vi "FPL-Compute FPL.vi"(0 "path in":path, 11 "error in (no error)":errorcluster) -> (4 "path out":path, 15 "error out":errorcluster)   [LabVIEW 2015]
uses:
  Utility VIs/Math VIs/Z to dB, degrees (1D).vi
panel:
  out "XY Graph":T1(graph)
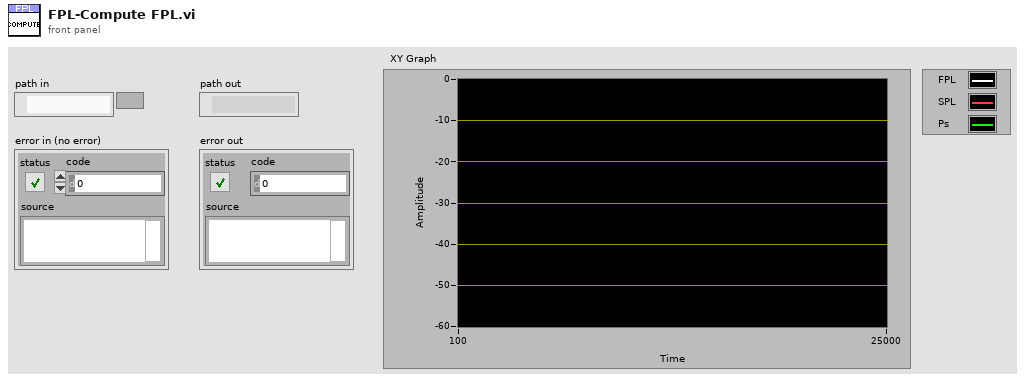
[diagram p1: front panel]
types:
  T1 = cluster{"Frequency (Hz)":dbl[], "Magnitude (dB)":dbl[]}[]
  T2 = cluster{"Frequency (Hz)":dbl[], "Magnitude (dB)":dbl[]}
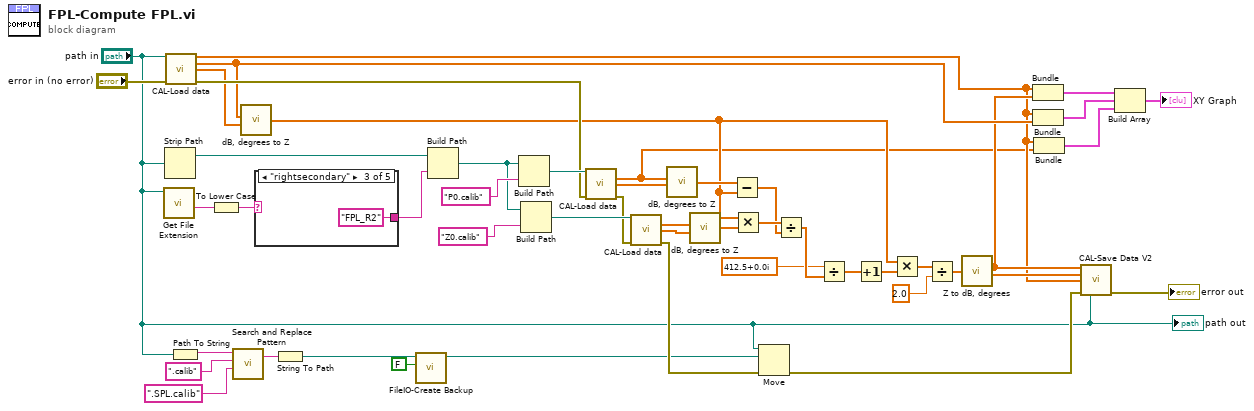
[diagram p0: block diagram]
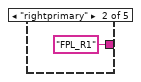
[diagram p3: hidden frame]
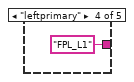
[diagram p4: hidden frame]
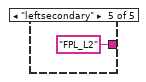
[diagram p5: hidden frame]
diagram:
  n1 = call <vilib>:"Get File Extension.vi"("file"="path in") -> ("filename without extension"=w48:string)  [unwired: 6 in, 4 out]
  n2 = Strip Path(path="path in") -> (stripped path=w46:path)  [unwired: 1 out]
  n3 = call "CAL-Load data.vi"("user path"="path in", "error in (no error)"="error in (no error)") -> ("Frequency (Hz)"=w4:dbl[], "Mag"=w18:dbl[], "Phase"=w33:dbl[], "error out"=w38:errorcluster)  [unwired: 6 in, 4 out]
  n4 = Path To String(path="path in") -> (string=w16:string)
  n5 = To Lower Case(string=w48) -> (all lower case string=w47:string)
  n6 = call <vilib>:"Search and Replace Pattern.vi"("string"=w16, "regular expression (\"\")"=".calib" ("regular expression (\"\")"), "replace string (\"\")"=".SPL.calib" ("regular expression (\"\")")) -> ("result string"=w13:string)  [unwired: 2 in, 1 out]
  n7 = call "dB, degrees to Z.vi"("Magnitude (dB)"=w18, "Phase (degrees)"=w33) -> ("Z"=w21:cdb[])  [unwired: 5 in]
  n8 = case shown="\"rightsecondary\"" w47 {
    tunnel: [_ "FPL_R1" "FPL_R2" "FPL_L1" "FPL_L2"] -> w45
    frame "", Default {
    }
    frame "rightprimary" {
    }
    frame "rightsecondary" {
    }
    frame "leftprimary" {
    }
    frame "leftsecondary" {
    }
  }
  n9 = String To Path(string=w13) -> (path=w7:path)
  n10 = call "FileIO-Create Backup.vi"("Delete tag"=FALSE, "Path"=w7) -> ("Path (thru)"=w6:path)  [unwired: 6 in, 3 out]
  n11 = Build Path(base path=w46, name or relative path=w45) -> (appended path=w43:path)
  n12 = Build Path(base path=w43, name or relative path="P0.calib") -> (appended path=w40:path)
  n13 = Build Path(base path=w43, name or relative path="Z0.calib") -> (appended path=w39:path)
  n14 = call "CAL-Load data.vi"("user path"=w40, "error in (no error)"=w38) -> ("Mag"=w3:dbl[], "Phase"=w36:dbl[], "error out"=w37:errorcluster)  [unwired: 6 in, 5 out]
  n15 = call "CAL-Load data.vi"("user path"=w39, "error in (no error)"=w37) -> ("Mag"=w35:dbl[], "Phase"=w34:dbl[], "error out"=w17:errorcluster)  [unwired: 6 in, 5 out]
  n16 = call "dB, degrees to Z.vi"("Magnitude (dB)"=w3, "Phase (degrees)"=w36) -> ("Z"=w32:cdb[])  [unwired: 5 in]
  n17 = call "dB, degrees to Z.vi"("Magnitude (dB)"=w35, "Phase (degrees)"=w34) -> ("Z"=w28:cdb[])  [unwired: 5 in]
  n18 = Subtract(x=w32, y=w21) -> (x-y=w30:cdb[])
  n19 = Multiply(x=w21, y=w28) -> (x*y=w31:cdb[])
  n20 = Move(source path="path in", error in=w17, 10:w6) -> (error out=w9:errorcluster)  [unwired: 2 in, 2 out]
  n21 = Divide(x=w31, y=w30) -> (x/y=w29:cdb[])
  n22 = Divide(x=cdb 412.5+0.0i, y=w29) -> (x/y=w27:cdb[])
  n23 = Increment(x=w27) -> (x+1=w26:cdb[])
  n24 = Multiply(x=w21, y=w26) -> (x*y=w25:cdb[])
  n25 = Divide(x=w25, y=2.0) -> (x/y=w23:cdb[])
  n26 = call-poly "Z to dB, degrees.vi"("Z"=w23) -> ("Magnitude (dB)"=w12:dbl[], "Phase (degrees)"=w11:dbl[])  [unwired: 5 in]
  n27 = Bundle("Frequency (Hz)"=w4, "Magnitude (dB)"=w12) -> (w22:T2)  [unwired: 1 in]
  n28 = Bundle("Frequency (Hz)"=w4, "Mag"=w18) -> (w19:cluster{"Frequency (Hz)":dbl[], "Mag":dbl[]})  [unwired: 1 in]
  n29 = Bundle("Frequency (Hz)"=w4, "Mag"=w3) -> (w2:cluster{"Frequency (Hz)":dbl[], "Mag":dbl[]})  [unwired: 1 in]
  n30 = call "CAL-Save Data V2.vi"("Mag"=w12, "Phase"=w11, "Frequency"=w4, "error in (no error)"=w9, "path"="path in") -> ("error out"=→"error out":errorcluster)  [unwired: 9 in, 1 out]
  n31 = Build Array(w22, w19, w2) -> (→"XY Graph":cluster{"Frequency (Hz)":dbl[], "Mag":dbl[]}[])
  "path out" <- "path in"
